vi "párbeszédablakok.vi"(11 "kezelõpult":T1={"Filt_alsó"=750.0, "Filt_felsõ"=7400.0, "Optikai elem hossza (km)"=0.000445, "Referencia hullámhossz (nm)"=800.0, " Illesztendõ polinom fokszáma"=7, "Megjegyzések"=""}) -> ()   [LabVIEW 2016]
doc: "A kezelõpult monitorozása és a felhasználó értésítése nem megfelelõ értékek beírása esetén."
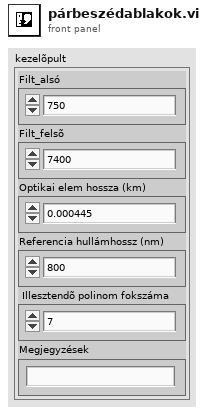
[diagram p1: front panel]
types:
  T1 = typedef "kezelõpult.ctl" = cluster{"Filt_alsó":dbl, "Filt_felsõ":dbl, "Optikai elem hossza (km)":dbl, "Referencia hullámhossz (nm)":dbl, " Illesztendõ polinom fokszáma":i32, "Megjegyzések":string}
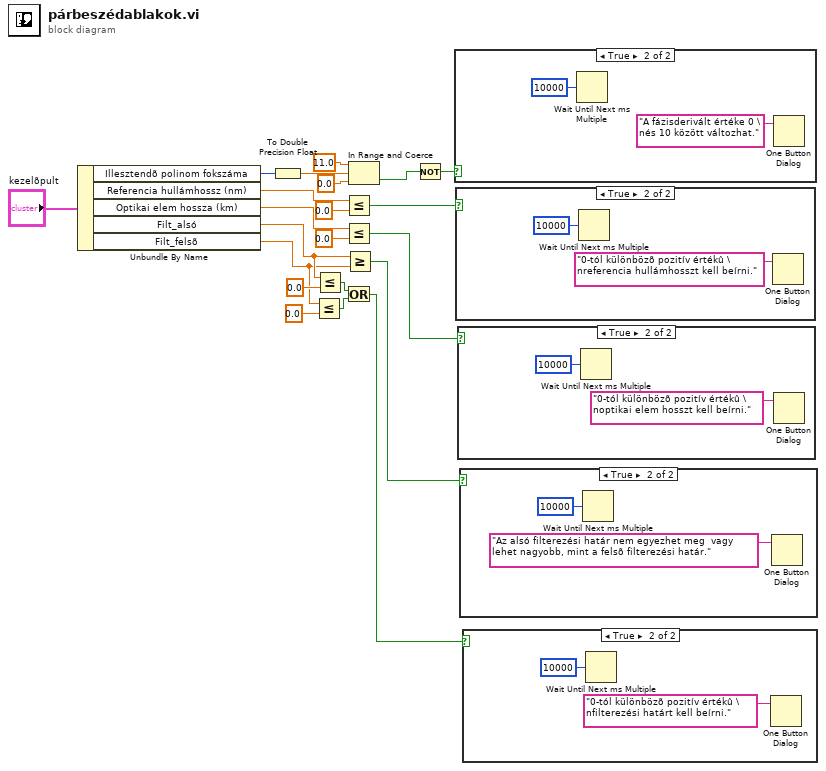
[diagram p0: block diagram]
diagram:
  n1 = Unbundle By Name("kezelõpult") -> ("Illesztendõ polinom fokszáma"=w15:i32, "Referencia hullámhossz (nm)"=w18:dbl, "Optikai elem hossza (km)"=w20:dbl, "Filt_alsó"=w8:dbl, "Filt_felsõ"=w7:dbl)
  n2 = To Double Precision Float(number=w15) -> (double precision float=w3:dbl)
  n3 = Less Or Equal?(x=w7, y=0.0) -> (x <= y?=w10:bool)
  n4 = Less Or Equal?(x=w8, y=0.0) -> (x <= y?=w9:bool)
  n5 = Less Or Equal?(x=w18, y=0.0) -> (x <= y?=w21:bool)
  n6 = Less Or Equal?(x=w20, y=0.0) -> (x <= y?=w14:bool)
  n7 = Or(x=w9, y=w10) -> (x .or. y?=w6:bool)
  n8 = Greater Or Equal?(x=w8, y=w7) -> (x >= y?=w13:bool)
  n9 = In Range and Coerce(upper limit=11.0, x=w3, lower limit=0.0) -> (In Range?=w1:bool)  [unwired: 1 out]
  n10 = Not(x=w1) -> (.not. x?=w2:bool)
  n11 = case shown="True" w2 {
    frame False {
    }
    frame True {
      n12 = Wait Until Next ms Multiple(millisecond multiple=u32 10000 ("milliseconds to wait")) -> ()  [unwired: 1 out]
      n13 = One Button Dialog(message="A fázisderivált értéke 0 \nés 10 között változhat.") -> ()  [unwired: 1 in, 1 out]
    }
  }
  n14 = case shown="True" w21 {
    frame False {
    }
    frame True {
      n15 = Wait Until Next ms Multiple(millisecond multiple=u32 10000 ("milliseconds to wait")) -> ()  [unwired: 1 out]
      n16 = One Button Dialog(message="0-tól különbözõ pozitív értékû \nreferencia hullámhosszt kell beírni.") -> ()  [unwired: 1 in, 1 out]
    }
  }
  n17 = case shown="True" w14 {
    frame False {
    }
    frame True {
      n18 = Wait Until Next ms Multiple(millisecond multiple=u32 10000 ("milliseconds to wait")) -> ()  [unwired: 1 out]
      n19 = One Button Dialog(message="0-tól különbözõ pozitív értékû \noptikai elem hosszt kell beírni.") -> ()  [unwired: 1 in, 1 out]
    }
  }
  n20 = case shown="True" w13 {
    frame False {
    }
    frame True {
      n21 = Wait Until Next ms Multiple(millisecond multiple=u32 10000 ("milliseconds to wait")) -> ()  [unwired: 1 out]
      n22 = One Button Dialog(message="Az alsó filterezési határ nem egyezhet meg  vagy lehet nagyobb, mint a felsõ filterezési határ.") -> ()  [unwired: 1 in, 1 out]
    }
  }
  n23 = case shown="True" w6 {
    frame False {
    }
    frame True {
      n24 = Wait Until Next ms Multiple(millisecond multiple=u32 10000 ("milliseconds to wait")) -> ()  [unwired: 1 out]
      n25 = One Button Dialog(message="0-tól különbözõ pozitív értékû \nfilterezési határt kell beírni.") -> ()  [unwired: 1 in, 1 out]
    }
  }
